vi "Write Nb Channel.vi"(8 "error in (no error)":errorcluster, 10 "Nb Channel":u16, 11 "Class LED Analyser FEASA in":refnum<class "Class LED Analyser FEASA.lvclass">) -> (0 "error out":errorcluster, 3 "Class LED Analyser FEASA out":refnum<class "Class LED Analyser FEASA.lvclass">)   [LabVIEW 2020, in "Library Instrument & Equipement.lvlib" / "Library LED Analyser.lvlib" / "Class LED Analyser FEASA.lvclass"]
uses:
  Class LED Analyser FEASA.lvclass
  Class LED Analyser FEASA.lvclass/Class LED Analyser FEASA.ctl
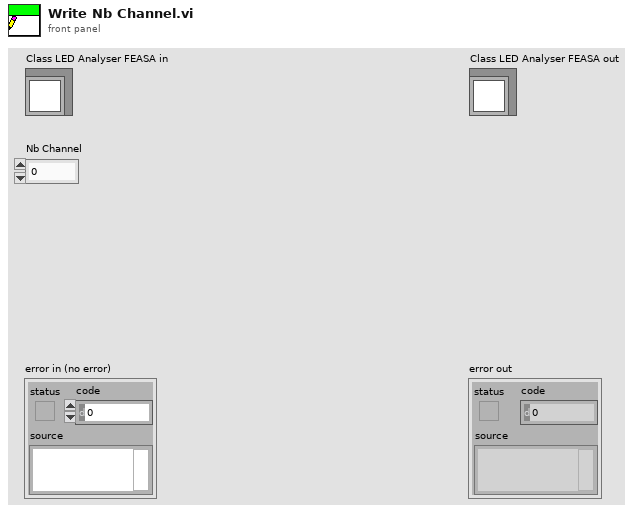
[diagram p1: front panel]
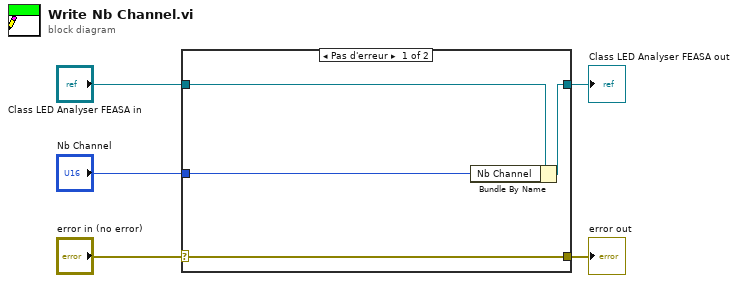
[diagram p0: block diagram]
diagram:
  n1 = case shown="Pas d'erreur" "error in (no error)" {
    selector: "error in (no error)" -> [w9 w10]
    tunnel: [w9 w10] -> w4
    tunnel: [w7 w11] -> w2
    tunnel: "Class LED Analyser FEASA in" -> [w8 w11]
    tunnel: "Nb Channel" -> [w6 _]
    frame No Error {
      n2 = Bundle By Name(cluster=w8, "Nb Channel"=w6) -> (w7:refnum<class "Class LED Analyser FEASA.lvclass">)
    }
    frame Error {
    }
  }
  "error out" <- w4
  "Class LED Analyser FEASA out" <- w2
